vi "Test Report Contain Failure Type.vi"(8 "error in (no error)":errorcluster, 11 "XML Report Test in":refnum<class "XML Report Test.lvclass">) -> (0 "error out":errorcluster, 3 "XML Report Test out":refnum<class "XML Report Test.lvclass">)   [LabVIEW 2020, in "XML Report Test.lvclass"]
uses:
  XML Report Test.lvclass
  XML Report Test.lvclass/XML Report Test.ctl
  source/Plugins/XML Report/XML Report.lvclass
  Test Doubles/Test Case Test Double/Methods.ctl
  Test Doubles/Test Case Test Double/Test Case Test Double.lvclass
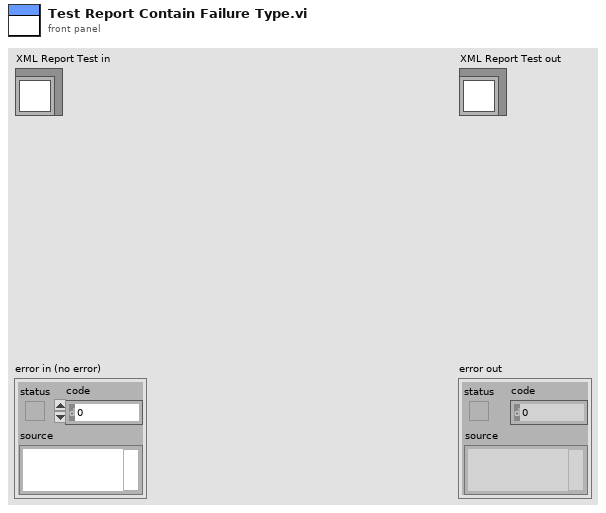
[diagram p1: front panel]
types:
  T1 = typedef "Test Case Test Double.lvclass/Methods.ctl" = enum16{"Test Failing Test.vi", "Test Passing Test.vi", "Test Error Test.vi", "Test Skip Test.vi", "Test Passing Pass If Test.vi", "Test Failing Pass If Test.vi", "Test Failing Fail If Test.vi", "Test Passing Fail If Test.vi", "Test Passing Pass If Error Test.vi", "Test Failing Pass If Error Test.vi", "Test Passing Fail If Error Test.vi", "Test Failing Fail If Error Test.vi", "Test Passing Pass If Equal Test.vi", "Test Failing Pass If Equal Test.vi", "Test Failing Fail If Equal Test.vi", "Test Passing Fail If Equal Test.vi", "Freezing Test.vi"}
  T2 = typedef "Result.lvlib/Result.ctl" = cluster{"Name":string, "Message":string, "Description":string, "Status":T3, "Result Type":T4, "Execution Time":dbl}
  T3 = typedef "Result.lvlib/Status.ctl" = enum16{"", "Passed", "Failed", "Error", "Skipped", "Setup Error", "Broken", "Teardown Error"}
  T4 = typedef "Result.lvlib/Type.ctl" = enum16{"Method", "Case", "Suite", "Pass", "Fail", "Skip", "Pass if", "Fail if", "Pass if Error", "Fail if Error", "Pass if Equal", "Fail if Equal"}
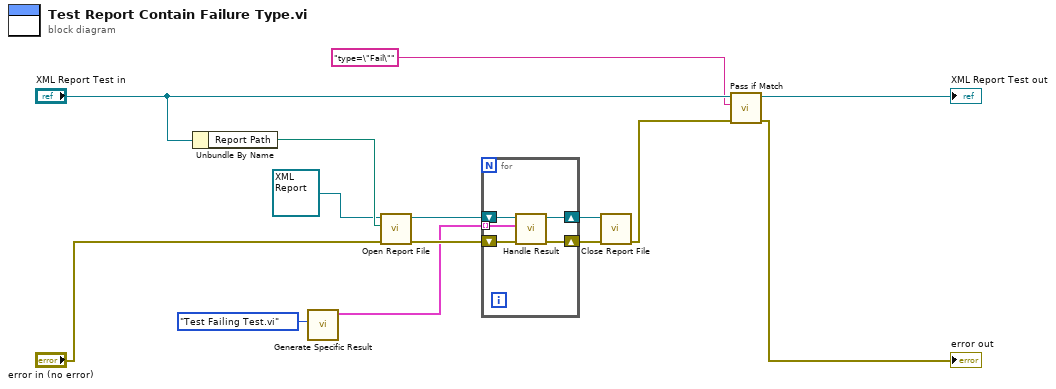
[diagram p0: block diagram]
diagram:
  n1 = Unbundle By Name("XML Report Test in") -> ("Report Path"=w8:path)
  n2 = call "Generate Specific Result.vi"("Test Method"=Methods."Test Failing Test.vi") -> ("Data"=w2:T2[])  [unwired: 9 in, 1 out]
  n3 = call-dynamic "Open Report File.vi"("error in (no error)"="error in (no error)", "Report Path"=w8, "XML Report In"=refnum<class "XML Report.lvclass"> refnum) -> ("error out"=w14:errorcluster, "XML Report Out"=w4:refnum<class "XML Report.lvclass">)  [unwired: 7 in]
  n4 = for {
    tunnel: w2 -> [w15] mode=indexing
    shift-right: [w18] -> w5
    shift-left: w14 -> [w19]
    shift-right: [w16] -> w3
    shift-left: w4 -> [w17]
    n5 = call-dynamic "Handle Result.vi"("error in (no error)"=w19, "Result"=w15, "XML Report In"=w17) -> ("error out"=w18:errorcluster, "XML Report Out"=w16:refnum<class "XML Report.lvclass">)  [unwired: 7 in]
  }
  n6 = call-dynamic "Close Report File.vi"("error in (no error)"=w5, "XML Report In"=w3) -> ("error out"=w10:errorcluster)  [unwired: 9 in]
  n7 = call "Pass if Match.vi"("error in (no error)"=w10, "regular expression"="type=\"Fail\"", "XML Report Test in"="XML Report Test in") -> ("error out"=→"error out":errorcluster, "XML Report Test out"=→"XML Report Test out":refnum<class "XML Report Test.lvclass">)  [unwired: 6 in, 1 out]
